vi "BUILD_install upload.vi"() -> ()   [LabVIEW 2013]
panel:
  in  "buildlog":path
  out "error out":errorcluster
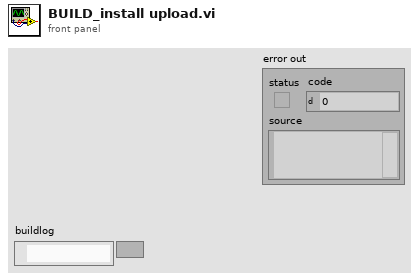
[diagram p1: front panel]
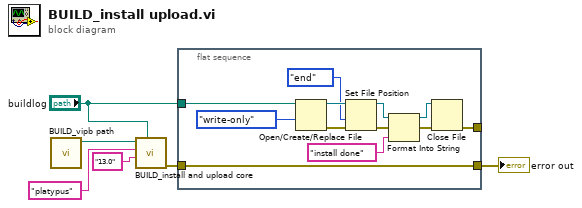
[diagram p0: block diagram]
diagram:
  n1 = call "BUILD_vipb path.vi"() -> ("appended path"=w4:path)  [unwired: 11 in]
  n2 = call "BUILD_install and upload core.vi"("buildlog"="buildlog", "LabVIEW Version"="13.0", "Repository Name"="platypus", "appended path"=w4) -> ("error out"=w2:errorcluster)  [unwired: 7 in]
  n3 = flat-sequence {
    tunnel: [w10] -> _
    tunnel: [w9] -> w3
    tunnel: w2 -> [w9]
    tunnel: "buildlog" -> [w7]
    frame #0 {
      n4 = Open/Create/Replace File(file path (use dialog)=w7, access (0:read/write)=enum16{"read/write", "read-only", "write-only"}."write-only") -> (refnum out=w18:refnum<file>, error out=w17:errorcluster)  [unwired: 4 in, 1 out]
      n5 = Set File Position(refnum=w18, from (0:start)=enum16{"start", "end", "current"}."end", error in=w17) -> (refnum out=w16:refnum<file>, error out=w15:errorcluster)  [unwired: 1 in]
      n6 = Format Into String(initial string=w16, error in=w15, "install done") -> (resulting string=w14:refnum<file>, error out=w13:errorcluster)  [unwired: 1 in]
      n7 = Close File(refnum=w14, error in=w13) -> (error out=w10:errorcluster)  [unwired: 1 out]
    }
  }
  "error out" <- w3
